vi "Stuck_Alarm.vi"(1 "Time Target (s)":dbl=5.0, 2 "Finish_Measurement":bool, 3 "Start_Measurement":bool) -> (0 "Stuck_Alarm":bool caption="Time has Elapsed")   [LabVIEW 2020]
doc: "Show off alarm during measurement if piece stuck in the middle."
panel:
  out "Elapsed Time (s)":dbl
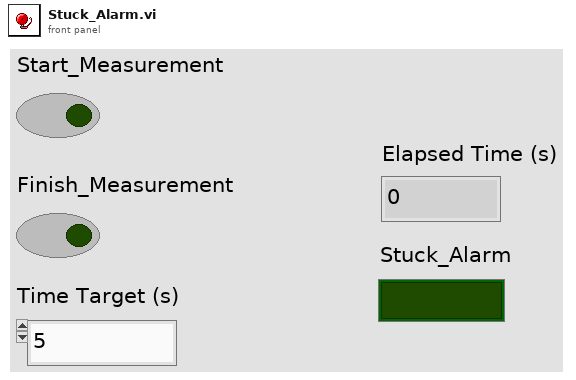
[diagram p1: front panel]
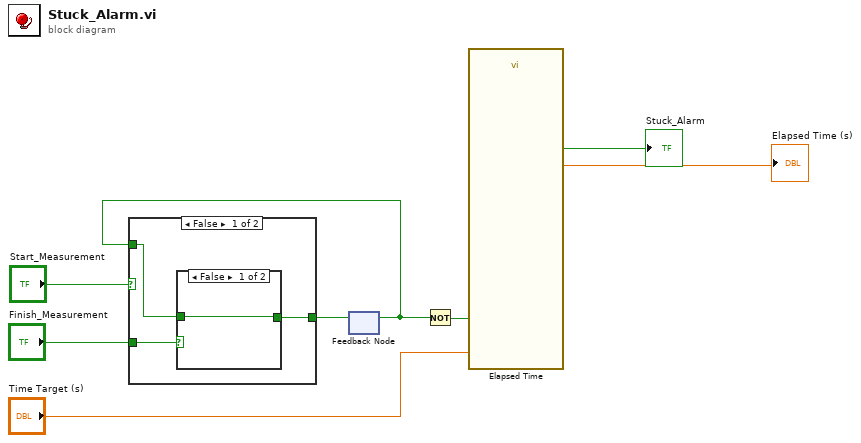
[diagram p0: block diagram]
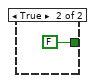
[diagram p2: hidden frame]
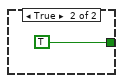
[diagram p3: hidden frame]
diagram:
  n1 = feedback #1() -> (w2:bool)  [unwired: 1 in]
  n2 = case shown="False" "Start_Measurement" {
    tunnel: [w10 TRUE] -> w5
    tunnel: "Finish_Measurement" -> [w11 _]
    tunnel: w2 -> [w9 _]
    frame False {
      n3 = case shown="False" w11 {
        tunnel: [w12 FALSE] -> w10
        tunnel: w9 -> [w12 _]
        frame False {
        }
        frame True {
        }
      }
    }
    frame True {
    }
  }
  n4 = feedback-in #1(w5) -> ()
  n5 = Not(x=w2) -> (.not. x?=w7:bool)
  n6 = call "Elapsed Time"("Time Target (s)"="Time Target (s)", "Reset"=w7) -> ("Elapsed Time (s)"=→"Elapsed Time (s)":dbl, "Time has Elapsed"=→"Stuck_Alarm":bool)  [unwired: 10 in, 6 out]
